vi "getADC.vi"(8 "error in (no error)":errorcluster, 10 "ILC In":refnum<class "ILC.lvclass">, 11 "ILCADC1 in":refnum<class "ILCADC1.lvclass">) -> (0 "error out":errorcluster, 1 "ADC Value":dbl[unit], 2 "ILC Out":refnum<class "ILC.lvclass">, 3 "ILCADC1 out":refnum<class "ILCADC1.lvclass">)   [LabVIEW 2015, in "ILCADC1.lvclass"]
uses:
  ILCADC1.lvclass
  <userlib>/Common/ILC/ILC/ILC.lvclass
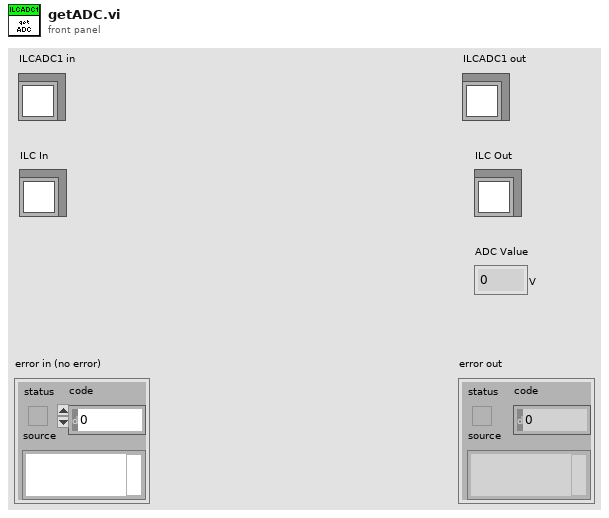
[diagram p1: front panel]
types:
  T1 = typedef "ILCCommon.lvlib/ILCTypedefs.lvlib/ADC Eng.ctl" = cluster{"Ch1":dbl[unit], "Ch2":dbl[unit], "Ch3":dbl[unit], "Ch4":dbl[unit]}
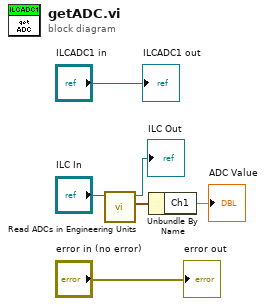
[diagram p0: block diagram]
diagram:
  n1 = call <userlib>:"Read ADCs in Engineering Units.vi"("ILC in"="ILC In") -> ("ADCs in Engineering Units"=w4:T1, "ILC out"=→"ILC Out":refnum<class "ILC.lvclass">)  [unwired: 9 in]
  n2 = Unbundle By Name(w4) -> ("Ch1"=→"ADC Value":dbl[unit])
  "error out" <- "error in (no error)"
  "ILCADC1 out" <- "ILCADC1 in"
